vi "rad_Apply Network Settings (Static).bak.vi"(6 "Timeout in ms (4s)":u32=4000, 8 "error in (no error)":errorcluster, 10 "Requested settings":T1={"Hostname"="", "Serial number"="", "Product name"="", "Product code"=0, "System status"="", "Credential type"=enum."None/Unlocked", "User added?"=FALSE, "Primary NIC"={"MAC address"="", "IP Address Request Mode"=2, "IP address"="", "Subnet mask"="", "Gateway"="", "DNS server"=""}} {"Primary NIC"."IP Address Request Mode" items=["Static"=1, "DHCP/Link-Local"=2, "Link-Local Only"=4, "DHCP Only"=8]}, 11 "Existing settings":T1={"Hostname"="", "Serial number"="", "Product name"="", "Product code"=0, "System status"="", "Credential type"=enum."None/Unlocked", "User added?"=FALSE, "Primary NIC"={"MAC address"="", "IP Address Request Mode"=2, "IP address"="", "Subnet mask"="", "Gateway"="", "DNS server"=""}} {"Primary NIC"."IP Address Request Mode" items=["Static"=1, "DHCP/Link-Local"=2, "Link-Local Only"=4, "DHCP Only"=8]}) -> (0 "error out":errorcluster, 3 "Target settings out":T1={"Hostname"="", "Serial number"="", "Product name"="", "Product code"=0, "System status"="", "Credential type"=enum."None/Unlocked", "User added?"=FALSE, "Primary NIC"={"MAC address"="", "IP Address Request Mode"=2, "IP address"="", "Subnet mask"="", "Gateway"="", "DNS server"=""}} {"Primary NIC"."IP Address Request Mode" items=["Static"=1, "DHCP/Link-Local"=2, "Link-Local Only"=4, "DHCP Only"=8]})   [LabVIEW 2013]
uses:
  TypeDefs/rad_Target Information.ctl
  TypeDefs/rad_Target Network Settings.ctl
  <vilib>/nisyscfg/Save Changes (System).vi
  <vilib>/nisyscfg/Close (System).vi
  <resource>/objmgr/nisysapi.rc
  <vilib>/nisyscfg/nisyscfg.lvlib
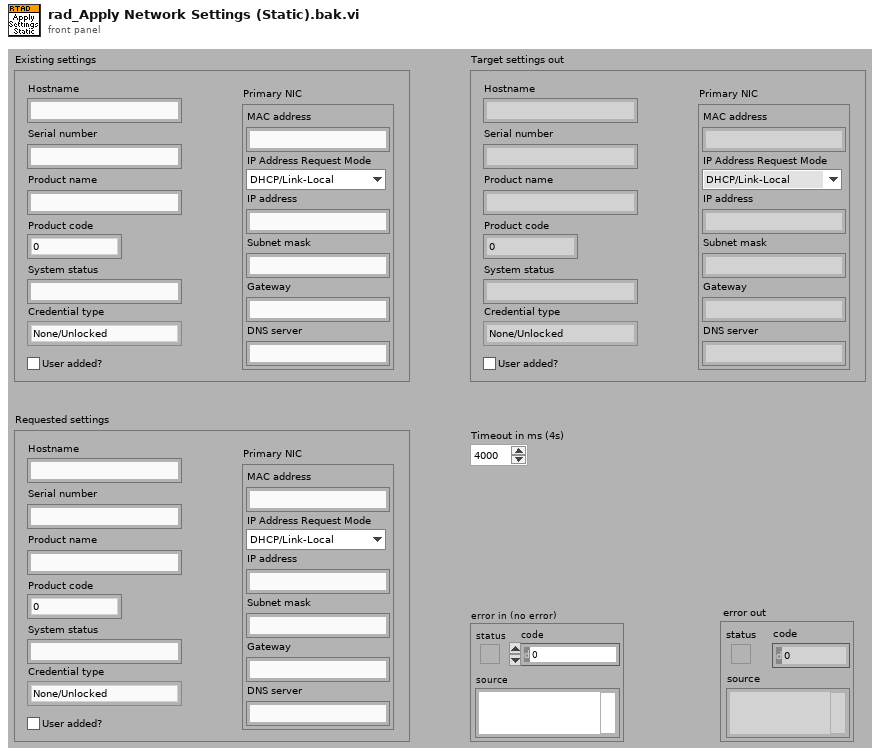
[diagram p1: front panel]
types:
  T1 = typedef "rad_Target Information.ctl" = cluster{"Hostname":string, "Serial number":string, "Product name":string, "Product code":i32, "System status":string, "Credential type":enum16{"None/Unlocked", "FTP Password", "NIAuth Credentials"}, "User added?":bool, "Primary NIC":T2}
  T2 = typedef "rad_Target Network Settings.ctl" = cluster{"MAC address":string, "IP Address Request Mode":i32, "IP address":string, "Subnet mask":string, "Gateway":string, "DNS server":string}
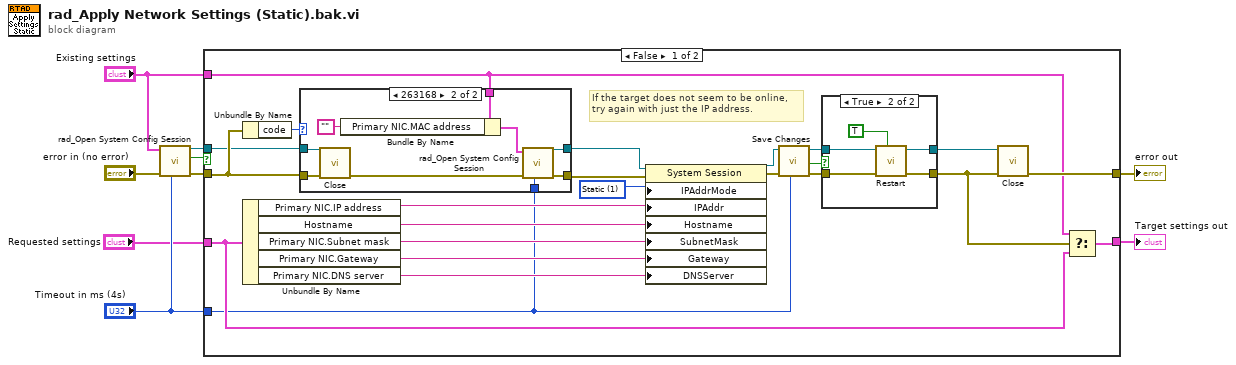
[diagram p0: block diagram]
diagram:
  n1 = call "rad_Open System Config Session.vi"("Timeout ms (4000)"="Timeout in ms (4s)", "error in (no error)"="error in (no error)", "Target settings"="Existing settings") -> ("error out"=w5:errorcluster, "Cancelled"=w4:bool, "Session out"=w7:refnum<k21>)  [unwired: 5 in, 1 out]
  n2 = case shown="False" w4 {
    tunnel: [w17 w51] -> w1
    tunnel: [w32 w52] -> w8
    tunnel: w7 -> [w10 _]
    tunnel: "Timeout in ms (4s)" -> [w15 _]
    tunnel: "Requested settings" -> [w18 _]
    tunnel: w5 -> [w11 w52]
    tunnel: "Existing settings" -> [w16 w51]
    frame False {
      w26 = 1 items=["Static"=1, "DHCP/Link-Local"=2, "Link-Local Only"=4, "DHCP Only"=8] ("Primary NIC:IP Address Request Mode")
      # "If the target does not seem to be online,\ntry again with just the IP address."
      n3 = Unbundle By Name(w11) -> ("code"=w12:i32)
      n4 = Unbundle By Name(w18) -> ("Primary NIC.IP address"=w31:string, "Hostname"=w30:string, "Primary NIC.Subnet mask"=w29:string, "Primary NIC.Gateway"=w28:string, "Primary NIC.DNS server"=w27:string)
      n5 = case shown="263168" w12 {
        tunnel: w11 -> [w33 w43]
        tunnel: w10 -> [w34 w42]
        tunnel: w16 -> [_ w41]
        tunnel: w15 -> [_ w37]
        tunnel: [w33 w36] -> w14
        tunnel: [w34 w35] -> w13
        frame Default {
        }
        frame 263168 {
          n6 = call-poly <vilib>:"Close.vi"("error in (no error)"=w43, "Session in"=w42) -> ("error out"=w38:errorcluster)  [unwired: 9 in]
          n7 = Bundle By Name(cluster=w41, "Primary NIC.MAC address"="") -> (w39:T1)
          n8 = call "rad_Open System Config Session.vi"("Timeout ms (4000)"=w37, "error in (no error)"=w38, "Target settings"=w39) -> ("error out"=w36:errorcluster, "Session out"=w35:refnum<k21>)  [unwired: 5 in, 2 out]
        }
      }
      n9 = property class="System Session"(reference=w13, error in=w14, "IPAddrMode"=w26, "IPAddr"=w31, "Hostname"=w30, "SubnetMask"=w29, "Gateway"=w28, "DNSServer"=w27) -> (reference out=w25:refnum<k21>, error out=w24:errorcluster)
      n10 = call-poly <vilib>:"Save Changes.vi"("Remote Timeout (300,000 ms)"=w15, "error in (no error)"=w24, "Session in"=w25) -> ("error out"=w22:errorcluster, "Changes Require Restart"=w23:bool, "Session out"=w21:refnum<k21>)  [unwired: 5 in, 1 out]
      n11 = case shown="True" w23 {
        tunnel: w22 -> [w45 w50]
        tunnel: [w45 w49] -> w19
        tunnel: w21 -> [w44 w48]
        tunnel: [w44 w47] -> w20
        frame False {
        }
        frame True {
          n12 = call <vilib>:"Restart.vi"("Wait Until Complete (T)"=TRUE ("wait until complete (T)"), "error in (no error)"=w50, "Session in"=w48) -> ("error out"=w49:errorcluster, "Session out"=w47:refnum<k21>)  [unwired: 6 in, 1 out]
        }
      }
      n13 = call-poly <vilib>:"Close.vi"("error in (no error)"=w19, "Session in"=w20) -> ("error out"=w32:errorcluster)  [unwired: 9 in]
      n14 = Select(t=w16, s=w19, f=w18) -> (s? t:f=w17:T1)
    }
    frame True {
    }
  }
  "error out" <- w8
  "Target settings out" <- w1
